vi "ConfigInstr.vi"(6 "InstrumentName":string, 7 "VisaRessIn":refnum<visa-resource-name>, 8 "error in (no error)":errorcluster caption="entrée d'erreur (pas d'erreur)", 9 "FirstClassInst":bool, 10 "Function":string, 11 "GenData In":refnum<class "LeafMagnetometer.lvclass"> caption="DNL_LabVIEW Object in") -> (0 "error out":errorcluster caption="sortie d'erreur", 3 "GenData Out":refnum<class "LeafMagnetometer.lvclass"> caption="DNL_LabVIEW Object out")   [LabVIEW 2019, in "LeafMagnetometer.lvclass"]
uses:
  LeafMagnetometer.lvclass
  C:/Programmes Labview/LabscanV1A/DevicesClass/BaseDevice/BaseDevice.lvclass
  LeafMagnetometer_Func.ctl
  LeafMagnetometer.lvclass/LeafMagnetometer.ctl
  BaseDevice/BaseDevice.lvclass/BaseDevice.ctl
  BaseDevice/Accessor/SetShowInstrNm.vi
panel:
  in  "DefaultDev_Func":T1
  out "VisaRessOut":refnum<visa-resource-name>
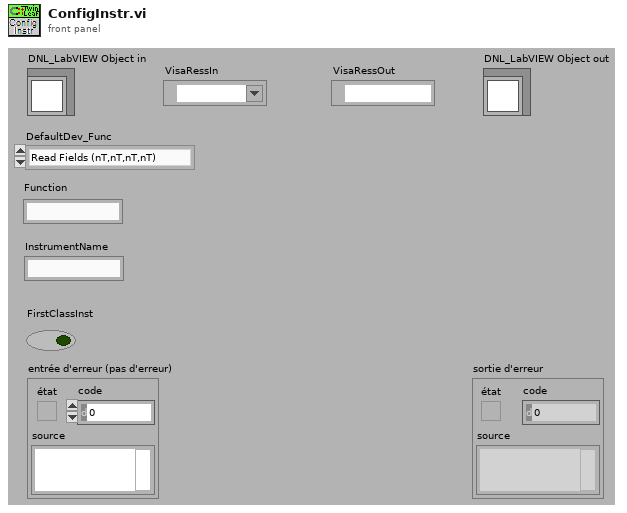
[diagram p1: front panel]
types:
  T1 = typedef "LeafMagnetometer.lvclass/LeafMagnetometer_Func.ctl" = enum16{"Read Fields (nT,nT,nT,nT)", "Read AVM Fields (nT)"}
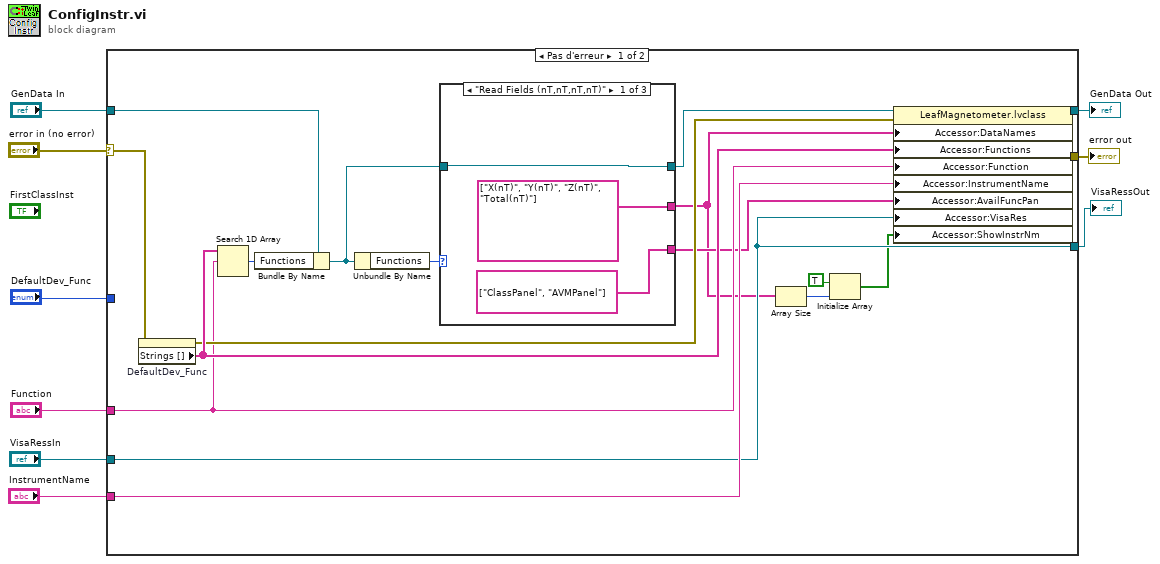
[diagram p0: block diagram]
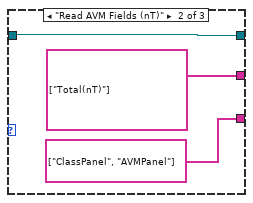
[diagram p2: hidden frame]
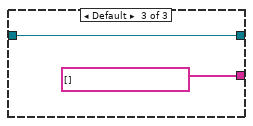
[diagram p3: hidden frame]
diagram:
  n1 = case shown="Pas d'erreur" "error in (no error)" {
    selector: "error in (no error)" -> [w21 w37]
    tunnel: [w27 w37] -> w8
    tunnel: "GenData In" -> [w22 w36]
    tunnel: [w26 w36] -> w6
    tunnel: "DefaultDev_Func" -> [_ _]
    tunnel: "Function" -> [w17 _]
    tunnel: "InstrumentName" -> [w16 _]
    tunnel: "VisaRessIn" -> [w14 _]
    tunnel: [w14 _] -> w1
    frame No Error {
      n2 = property on="DefaultDev_Func" class="Énum (strict)"(error in=w21) -> (error out=w20:errorcluster, "Strings []"=w24:string[])  [unwired: 1 in, 1 out]
      n3 = Search 1D Array(1D array=w24, element=w17) -> (index of element=w23:i32)  [unwired: 1 in]
      n4 = Bundle By Name(cluster=w22, "Functions"=w23) -> (w19:refnum<class "LeafMagnetometer.lvclass">)
      n5 = Unbundle By Name(w19) -> ("Functions"=w25:T1)
      n6 = case shown="\"Read Fields (nT,nT,nT,nT)\"" w25 {
        tunnel: [string[] ["X(nT)", "Y(nT)", "Z(nT)", "Total(nT)"] string[] ["Total(nT)"] string[] []] -> w11
        tunnel: w19 -> [w30 w33 w34]
        tunnel: [w30 w33 w34] -> w18
        tunnel: [string[] ["ClassPanel", "AVMPanel"] string[] ["ClassPanel", "AVMPanel"] _] -> w15
        frame "Read Fields (nT,nT,nT,nT)" {
        }
        frame "Read AVM Fields (nT)" {
        }
        frame Default {
        }
      }
      n7 = Array Size(array=w11) -> (size(s)=w13:i32)
      n8 = Initialize Array(TRUE, w13) -> (w10:bool[])
      n9 = property class="LeafMagnetometer.lvclass"(reference=w18, error in=w20, "Accessor:DataNames"=w11, "Accessor:Functions"=w24, "Accessor:Function"=w17, "Accessor:InstrumentName"=w16, "Accessor:AvailFuncPan"=w15, "Accessor:VisaRes"=w14, "Accessor:ShowInstrNm"=w10) -> (reference out=w26:refnum<class "LeafMagnetometer.lvclass">, error out=w27:errorcluster)
    }
    frame Error {
    }
  }
  "error out" <- w8
  "GenData Out" <- w6
  "VisaRessOut" <- w1
